vi "Encode_Float1616.vi"(1 ":16:16":dbl[](array[numeric])) -> (0 "Little Endian":u8[](array[numeric]))   [LabVIEW 2015, in "navX Library v3.lvlib" / "navX Registry Cache.lvclass"]
uses:
  navX Registry Cache.lvclass
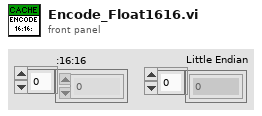
[diagram p1: front panel]
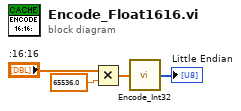
[diagram p0: block diagram]
diagram:
  n1 = Multiply(x=":16:16", y=65536.0) -> (x*y=w2:dbl[])
  n2 = call "Encode_Int32.vi"("Int32"=w2) -> ("Little Endian"=→"Little Endian":u8[])
